vi "Read Last Waveforms.vi"(8 "error in (no error)":errorcluster, 11 "Thermometer DAQmx in":refnum<class "Thermometer DAQmx.lvclass">) -> (0 "error out":errorcluster, 2 "Last Waveforms":map{u8, waveform(dbl)}(c390), 3 "Thermometer DAQmx out":refnum<class "Thermometer DAQmx.lvclass">)   [LabVIEW 2023, in "Thermometer.lvlib" / "Thermometer DAQmx.lvlib" / "Thermometer DAQmx.lvclass"]
uses:
  Thermometer DAQmx.lvclass
  Thermometer DAQmx.lvclass/Thermometer DAQmx.ctl
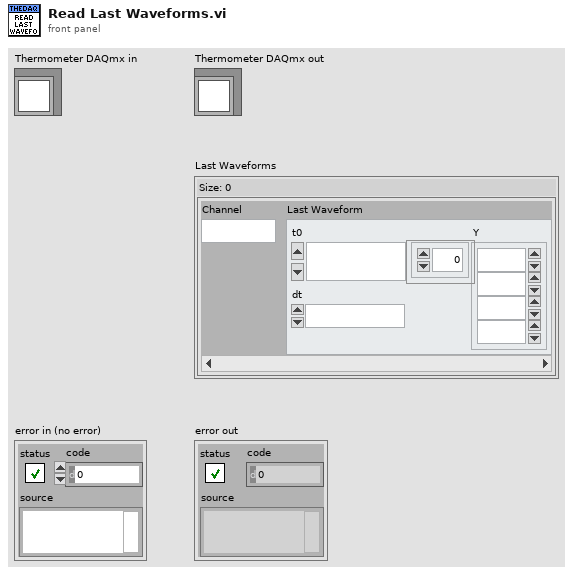
[diagram p1: front panel]
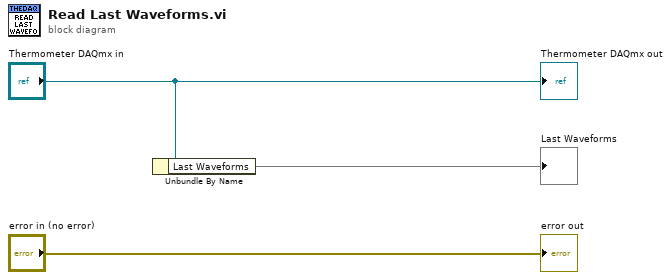
[diagram p0: block diagram]
diagram:
  n1 = Unbundle By Name("Thermometer DAQmx in") -> ("Last Waveforms"=→"Last Waveforms":map{u8, waveform(dbl)})
  "error out" <- "error in (no error)"
  "Thermometer DAQmx out" <- "Thermometer DAQmx in"
